vi "Read Private Info.vi"(11 "Executioner in":refnum<class "Executioner.lvclass">) -> (1 "Found?":bool, 3 "Info":string)   [LabVIEW 2017, in "Test Executive.lvlib" / "Executioner.lvclass"]
uses:
  <vilib>/gpm_packages/@cs/test-executive/Source/Test Executive/Executioner/Executioner.lvclass
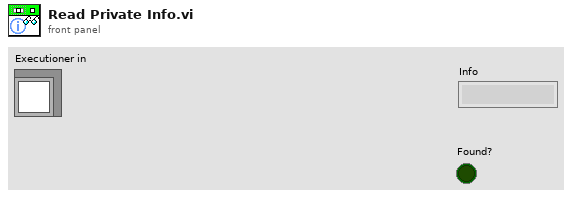
[diagram p1: front panel]
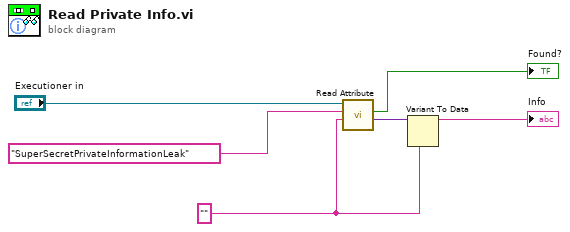
[diagram p0: block diagram]
diagram:
  w1 = ""
  n1 = call <vilib>:"Read Attribute.vi"("Type"=w1, "Name"="SuperSecretPrivateInformationLeak" ("Attribute Name"), "Executioner in"="Executioner in") -> ("Value"=w4:variant, "Found?"=→"Found?":bool)  [unwired: 6 in, 1 out]
  n2 = Variant To Data(type=w1, Variant=w4) -> (data=→"Info":string)  [unwired: 1 in, 1 out]
